vi "InitializeCmd_AToF.vi"(11 "BNC Control Queue in":refnum<queue>) -> ()   [LabVIEW 2013]
uses:
  Hardware/BNC(QuantumComposers)/BNC_States.ctl
  InitializationParams_BNC565_2Ch_AToF.ctl
  Hardware/BNC(QuantumComposers)/Command/Set C-Input.ctl
  Hardware/BNC(QuantumComposers)/Command/Set C-Mode.ctl
  Hardware/BNC(QuantumComposers)/Command/Set C-Output.ctl
  Hardware/BNC(QuantumComposers)/Command/Set C-Enable.ctl
panel:
  in  "BNC_Config":T6={"System"={"Rep.Rate"=1000.0, "Sys Ext Mode"=enum."Triggered", "Mode"=enum."Single Shot"}, "Channels"=[{"C-Input"={"Channel"=1, "Sync Source"=0}, "C-Mode"={"Channel"=1, "Delay"=0.0, "Width"=5e-06}, "C-Output"={"Channel"=1, "Polarity"=TRUE}, "C-Enables"={"Channel"=1, "Enable"=TRUE}}, {"C-Input"={"Channel"=2, "Sync Source"=0}, "C-Mode"={"Channel"=2, "Delay"=0.0, "Width"=2e-06}, "C-Output"={"Channel"=2, "Polarity"=TRUE}, "C-Enables"={"Channel"=2, "Enable"=TRUE}}]}
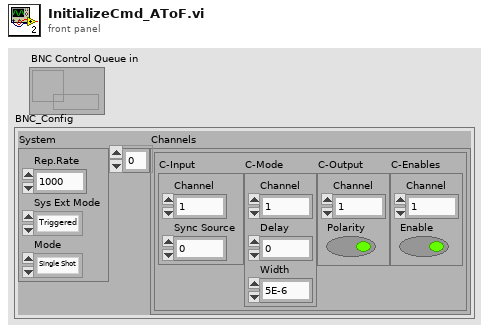
[diagram p1: front panel]
types:
  T1 = typedef "InitializationParams_BNC565_2Ch_AToF.ctl" = cluster{"C-Input":T2, "C-Mode":T3, "C-Output":T4, "C-Enables":T5}[]
  T2 = typedef "Set C-Input.ctl" = cluster{"Channel":i32, "Sync Source":i32}
  T3 = typedef "Set C-Mode.ctl" = cluster{"Channel":i32, "Delay":dbl, "Width":dbl}
  T4 = typedef "Set C-Output.ctl" = cluster{"Channel":i32, "Polarity":bool}
  T5 = typedef "Set C-Enable.ctl" = cluster{"Channel":i32, "Enable":bool}
  T6 = cluster{"System":cluster{"Rep.Rate":dbl, "Sys Ext Mode":enum16{"Disabled", "Triggered", "Gated", "Triggered & Gated"}, "Mode":enum16{"Normal", "Single Shot", "Duty Cycle", "Burst"}}, "Channels":T1}
  T7 = typedef "BNC_States.ctl" = cluster{"State":enum16{"Initialize", "Set System", "Set C-Input", "Set C-Mode", "Set C-Output", "Set C-Enable", "Manl_Trig", "Run", "Stop", "Query C Number", "Close", "Quit"}, "Para.":variant}
  T8 = cluster{"Rep.Rate":dbl, "Sys Ext Mode":enum16{"Disabled", "Triggered", "Gated", "Triggered & Gated"}, "Mode":enum16{"Normal", "Single Shot", "Duty Cycle", "Burst"}}
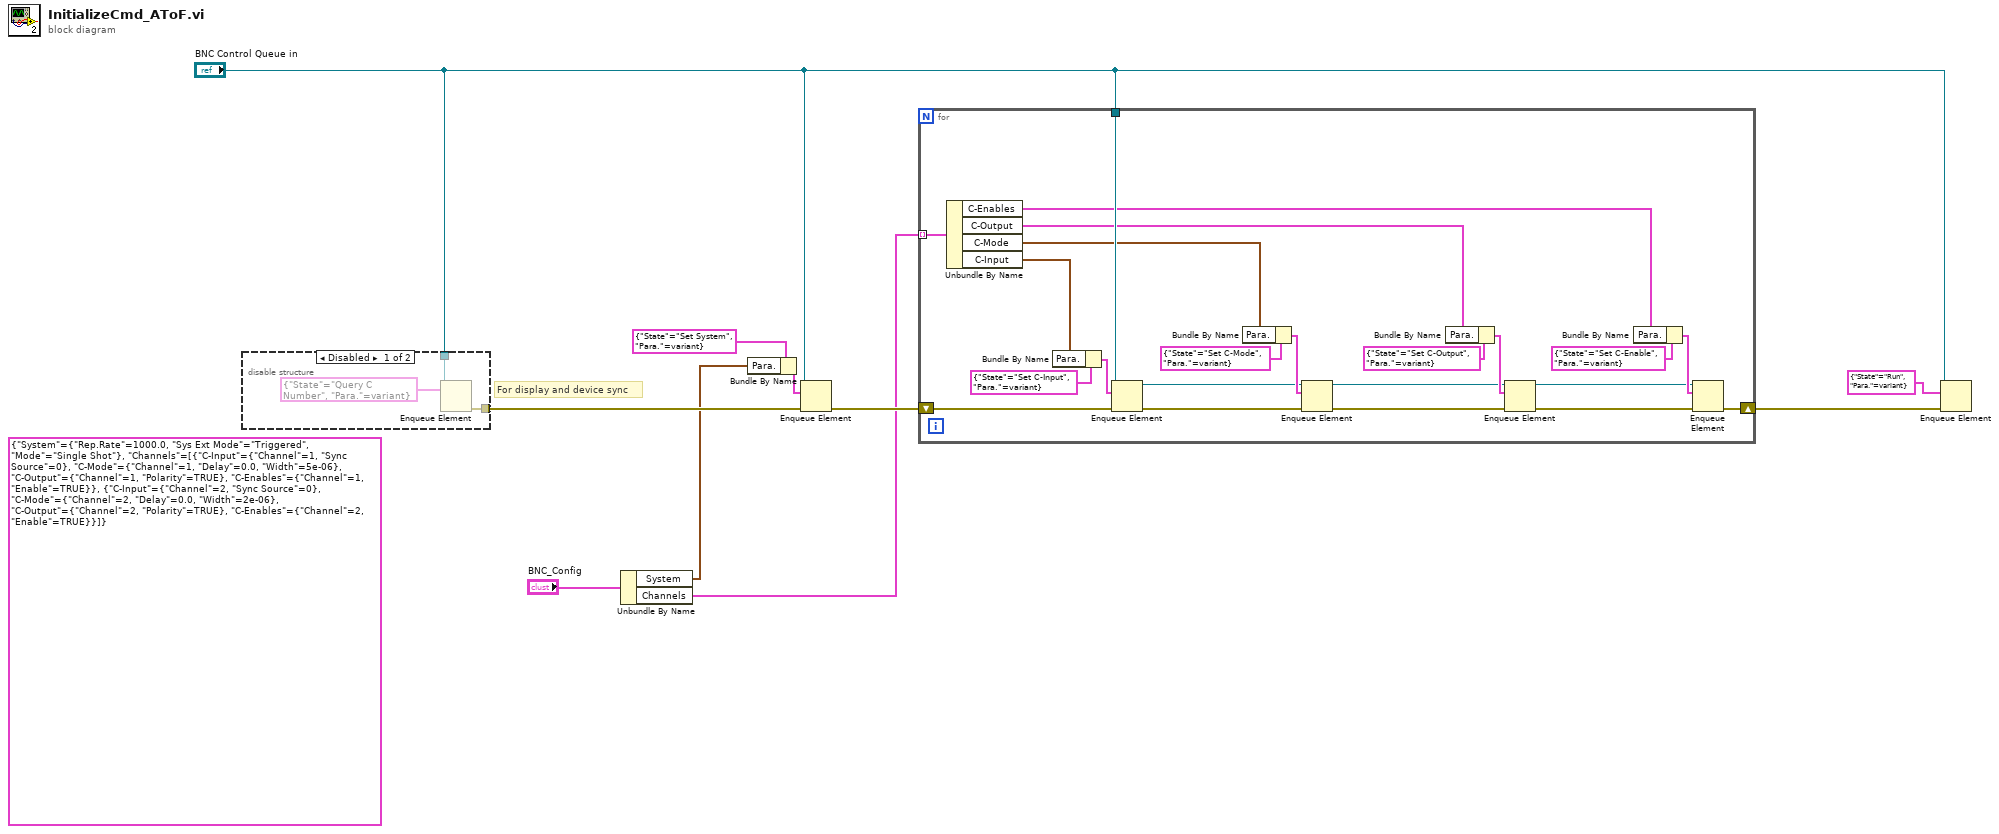
[diagram p0: block diagram]
diagram:
  (unwired) T6 {"System"={"Rep.Rate"=1000.0, "Sys Ext Mode"=enum."Triggered", "Mode"=enum."Single Shot"}, "Channels"=[{"C-Input"={"Channel"=1, "Sync Source"=0}, "C-Mode"={"Channel"=1, "Delay"=0.0, "Width"=5e-06}, "C-Output"={"Channel"=1, "Polarity"=TRUE}, "C-Enables"={"Channel"=1, "Enable"=TRUE}}, {"C-Input"={"Channel"=2, "Sync Source"=0}, "C-Mode"={"Channel"=2, "Delay"=0.0, "Width"=2e-06}, "C-Output"={"Channel"=2, "Polarity"=TRUE}, "C-Enables"={"Channel"=2, "Enable"=TRUE}}]}
  # "For display and device sync"
  n1 = disable-structure shown="Disabled" {
    disable-tunnel: [w13 _] -> w7
    disable-tunnel: "BNC Control Queue in" -> [w11 _]
    frame Disabled {
      n2 = Enqueue Element(queue=w11, element=T7 {"State"=enum."Query C Number", "Para."=variant}) -> (error out=w13:errorcluster)  [unwired: 2 in, 2 out]
    }
    frame Enabled {
    }
  }
  n3 = Unbundle By Name("BNC_Config") -> ("System"=w1:T8, "Channels"=w3:T1)
  n4 = Bundle By Name(cluster=T7 {"State"=enum."Set System", "Para."=variant} ("element"), "Para."=w1) -> (w9:T7)
  n5 = Enqueue Element(queue="BNC Control Queue in", element=w9, error in (no error)=w7) -> (error out=w10:errorcluster)  [unwired: 1 in, 2 out]
  n6 = for {
    tunnel: "BNC Control Queue in" -> [w32]
    tunnel: w3 -> [w31] mode=indexing
    shift-right: [w17] -> w6
    shift-left: w10 -> [w35]
    n7 = Unbundle By Name(w31) -> ("C-Enables"=w18:T5, "C-Output"=w19:T4, "C-Mode"=w20:T3, "C-Input"=w30:T2)
    n8 = Bundle By Name(cluster=T7 {"State"=enum."Set C-Input", "Para."=variant} ("element"), "Para."=w30) -> (w33:T7)
    n9 = Enqueue Element(queue=w32, element=w33, error in (no error)=w35) -> (queue out=w15:refnum<queue>, error out=w23:errorcluster)  [unwired: 1 in, 1 out]
    n10 = Bundle By Name(cluster=T7 {"State"=enum."Set C-Mode", "Para."=variant} ("element"), "Para."=w20) -> (w29:T7)
    n11 = Enqueue Element(queue=w15, element=w29, error in (no error)=w23) -> (queue out=w16:refnum<queue>, error out=w22:errorcluster)  [unwired: 1 in, 1 out]
    n12 = Bundle By Name(cluster=T7 {"State"=enum."Set C-Output", "Para."=variant} ("element"), "Para."=w19) -> (w26:T7)
    n13 = Enqueue Element(queue=w16, element=w26, error in (no error)=w22) -> (queue out=w14:refnum<queue>, error out=w21:errorcluster)  [unwired: 1 in, 1 out]
    n14 = Bundle By Name(cluster=T7 {"State"=enum."Set C-Enable", "Para."=variant} ("element"), "Para."=w18) -> (w25:T7)
    n15 = Enqueue Element(queue=w14, element=w25, error in (no error)=w21) -> (error out=w17:errorcluster)  [unwired: 1 in, 2 out]
  }
  n16 = Enqueue Element(queue="BNC Control Queue in", element=T7 {"State"=enum."Run", "Para."=variant}, error in (no error)=w6) -> ()  [unwired: 1 in, 3 out]
